vi "T7MOD_Write_FLOAT32_Registers.vi"(7 "FLOAT32 to Write":sgl[](array[numeric]), 8 "error in":errorcluster, 9 "Starting FLOAT32 Register":i32=55124, 10 "Remote Port":u16=502, 11 "Remote IP Address":string="192.168.1.15") -> (0 "error out":errorcluster, 1 "Written At":timestamp)   [LabVIEW 2018]
panel:
  # "Output"
  # "TCP Parameters"
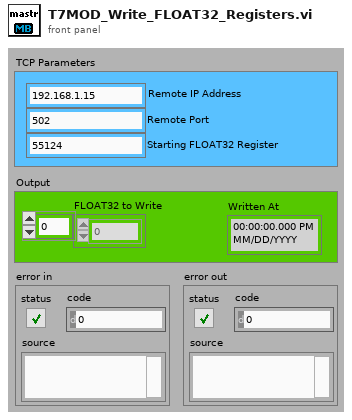
[diagram p1: front panel]
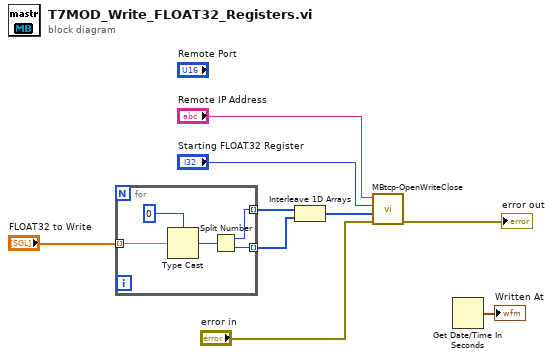
[diagram p0: block diagram]
diagram:
  n1 = for {
    tunnel: [w14] -> w8 mode=indexing
    tunnel: [w13] -> w7 mode=indexing
    tunnel: "FLOAT32 to Write" -> [w11] mode=indexing
    n2 = Type Cast(type=u32 0, x=w11) -> (*(type *) &x=w10:u32)
    n3 = Split Number(x=w10) -> (hi(x)=w13:u16, lo(x)=w14:u16)
  }
  n4 = Interleave 1D Arrays(w7, w8) -> (w3:u16[])
  n5 = call "MBtcp-OpenWriteClose.vi"("error in (no error)"="error in", "Values"=w3, "RegisterAddr"="Starting FLOAT32 Register", "IP Address(:port)"="Remote IP Address") -> ("error out"=→"error out":errorcluster)  [unwired: 7 in]
  n6 = Get Date/Time In Seconds() -> (seconds since 1Jan1904=→"Written At":timestamp)
